vi "SwitchConfiguration - Clear ListBoxes.vi"(8 "error in (no error)":errorcluster, 10 "ListBox 2 Ref In":refnum<vi>, 11 "ListBox 1 Ref In":refnum<vi>) -> (0 "error out":errorcluster, 2 "ListBox 2 Ref Out":refnum<vi>, 3 "ListBox 1 Ref Out":refnum<vi>)   [LabVIEW 2015, in "DMM-SWITCH-ScanList System Explorer.lvlib"]
uses:
  DMM-SWITCH-ScanList System Explorer.lvlib
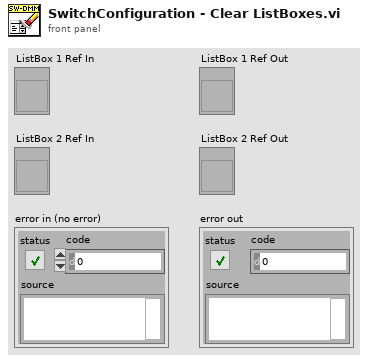
[diagram p1: front panel]
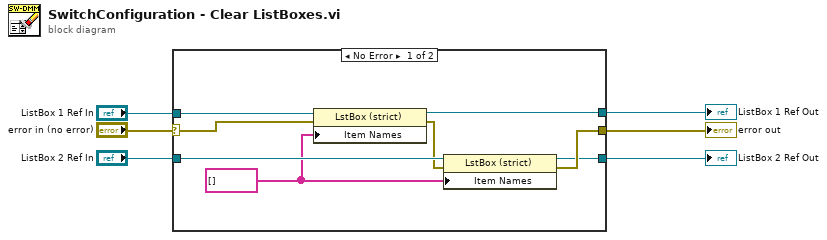
[diagram p0: block diagram]
diagram:
  n1 = case shown="No Error" "error in (no error)" {
    selector: "error in (no error)" -> [w7 w17]
    tunnel: [w14 w17] -> w6
    tunnel: "ListBox 1 Ref In" -> [w13 w16]
    tunnel: "ListBox 2 Ref In" -> [w12 w15]
    tunnel: [w9 w16] -> w3
    tunnel: [w8 w15] -> w2
    frame No Error {
      w10 = string[] [] ("Item Names")
      n2 = property class="LstBox (strict)"(reference=w13, error in=w7, "Item Names"=w10) -> (reference out=w9:refnum<vi>, error out=w11:errorcluster)
      n3 = property class="LstBox (strict)"(reference=w12, error in=w11, "Item Names"=w10) -> (reference out=w8:refnum<vi>, error out=w14:errorcluster)
    }
    frame Error {
    }
  }
  "error out" <- w6
  "ListBox 1 Ref Out" <- w3
  "ListBox 2 Ref Out" <- w2
